vi "Conditional Set of String.vi"(1 "set in":set{string}(c389)) -> (0 "Boolean":bool)   [LabVIEW 2020]
doc: "Monitors a set. The Data tab displays the size of the set and its contents. Use the Conditions tab to set a conditional breakpoint. You can set conditions based on the size of the set and/or its contents. If you select multiple conditions, LabVIEW executes a breakpoint if any of those conditions are true."
uses:
  46fe3144-eb06-4495-9ce8-2f4c16bfa097.vi
panel:
  in  "Tab Control":enum32{"Data   ", "Conditions      "}(tab)
  out "Set":set{string}(c389)
  in  "Does not contain a value":bool
  in  "Contains a value":bool
  in  "Number of Elements Condition":u16(ring) items=["Equal to", "Greater than", "Less than"]
  in  "Number of elements value":u32
  in  "Number of elements is":bool
  in  "Contains":string
  in  "Does Not Contain":string
  # "Pause if any of the following:"
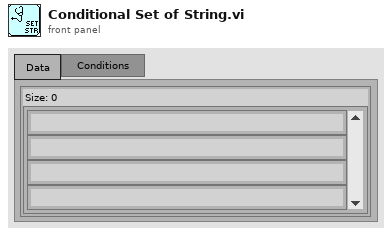
[diagram p1: front panel]
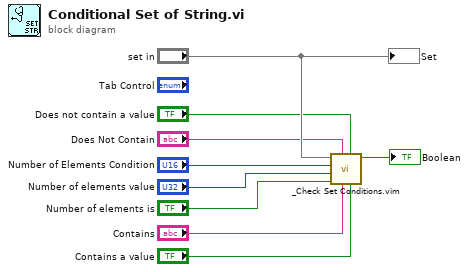
[diagram p0: block diagram]
diagram:
  n1 = call "_Check Set Conditions.vim"("Contains value"="Contains a value", "Does not contain value"="Does not contain a value", "contains"="Contains", "does not contain"="Does Not Contain", "# elements"="Number of elements is", "# elements value"="Number of elements value", "# elements condition"="Number of Elements Condition", "set"="set in") -> ("Pause"=→"Boolean":bool)  [unwired: 3 in]
  "Set" <- "set in"
